vi "Do Action.vi"(8 "error in (no error)":errorcluster, 11 "Encoder Drive Straight in":refnum<class "Encoder Drive Straight.lvclass">) -> (0 "error out":errorcluster, 3 "Encoder Drive Straight out":refnum<class "Encoder Drive Straight.lvclass">)   [LabVIEW 2016, in "Encoder Drive Straight.lvclass"]
uses:
  Encoder Drive Straight.lvclass
  Encoder Drive Straight.lvclass/Encoder Drive Straight.ctl
panel:
  out "Waveform Chart":cluster{"Distance":dbl, "Encoder Target":dbl}(graph)
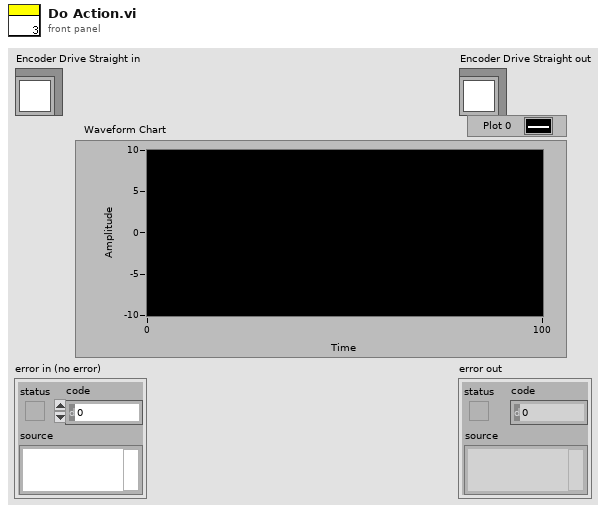
[diagram p1: front panel]
types:
  T1 = typedef "WPI_EncoderDevRef.ctl" = cluster{"DevStatus":errorcluster, "EncoderIndex":T2, "CounterIndex":T3, "DistancePerCount":dbl, "Decoding Type":T4}
  T2 = typedef "FPGA_EncoderIdx.ctl" = enum8{"Enc 0", "Enc 1", "Enc 2", "Enc 3", "Enc 4", "Enc 5", "Enc 6", "Enc 7", "Invalid"}
  T3 = typedef "FPGA_CounterCtrSystemIndex.ctl" = enum8{"Ctr 0", "Ctr 1", "Ctr 2", "Ctr 3", "Ctr 4", "Ctr 5", "Ctr 6", "Ctr 7", "Invalid"}
  T4 = typedef "WPI_EncoderType.ctl" = enum16{"1x", "2x", "4x"}
  T5 = typedef "WPI_RobotDriveDevRef.ctl" = cluster{"DevStatus":errorcluster, "Motors[]":T6[], "Square Inputs":bool, "Max Output":dbl}
  T6 = typedef "WPI_MotorControlDeviceRef.ctl" = cluster{"DeviceStatus":errorcluster, "Type":T7, "PWM":cluster{"PWM Channel":T8, "DeadBand":T9}, "CAN":cluster{"Device Number":u8, "SetOutput VI Ref":variant, "GetOutput VI Ref":variant, "Enable VI Ref":variant, "Disable VI Ref":variant, "Data":variant}, "Invert":bool}
  T7 = typedef "WPI_MotorControlType.ctl" = enum16{"PWM", "CAN"}
  T8 = typedef "FPGA_DIOPWMChannel.ctl" = enum8{"PWM 0", "PWM 1", "PWM 2", "PWM 3", "PWM 4", "PWM 5", "PWM 6", "PWM 7", "PWM 8", "PWM 9", "PWM MXP 0", "PWM MXP 1", "PWM MXP 2", "PWM MXP 3", "PWM MXP 4", "PWM MXP 5", "PWM MXP 6", "PWM MXP 7", "PWM MXP 8", "PWM MXP 9", "Invalid"}
  T9 = typedef "WPI_PWMDeadband.ctl" = cluster{"Name":string, "maxPositivePwm":i32, "minPositivePwm":i32, "centerPwm":i32, "maxNegativePwm":i32, "minNegativePwm":i32, "angularRange":u16}
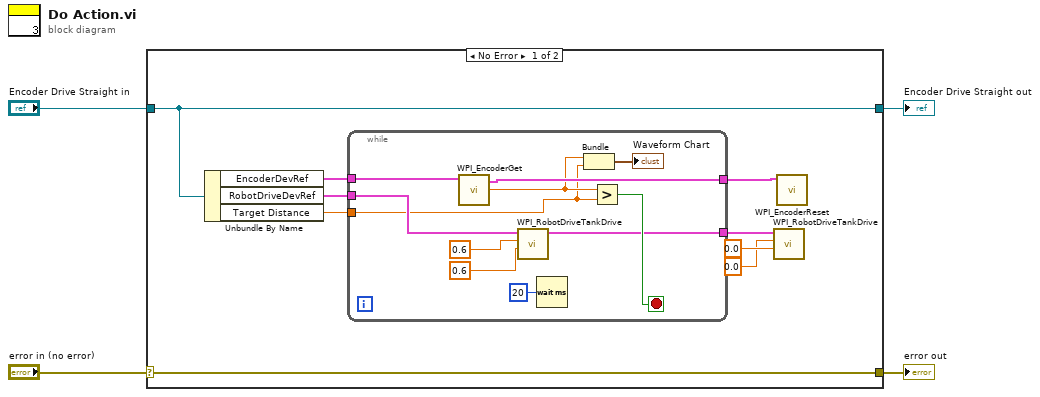
[diagram p0: block diagram]
diagram:
  n1 = case shown="No Error" "error in (no error)" {
    selector: "error in (no error)" -> [w13 w26]
    tunnel: [w13 w26] -> w3
    tunnel: [w12 w25] -> w1
    tunnel: "Encoder Drive Straight in" -> [w12 w25]
    frame No Error {
      n2 = Unbundle By Name(w12) -> ("EncoderDevRef"=w11:T1, "RobotDriveDevRef"=w10:T5, "Target Distance"=w5:dbl)
      n3 = while {
        tunnel: w11 -> [w24]
        tunnel: w10 -> [w23]
        tunnel: [w18] -> w9
        tunnel: [w17] -> w6
        tunnel: w5 -> [w14]
        stop <- w19 stop-if-true
        n4 = call <vilib>:"WPI_EncoderGet.vi"("EncoderDevRef"=w24) -> ("Distance"=w16:dbl, "EncoderDevRef"=w17:T1)  [unwired: 5 in, 4 out]
        n5 = call <vilib>:"WPI_RobotDriveTankDrive.vi"("Right axis value"=0.6, "Left axis value"=0.6, "RobotDriveDevRef"=w23) -> ("RobotDriveDevRef"=w18:T5)  [unwired: 6 in, 2 out]
        n6 = Wait (ms)(milliseconds to wait=u32 20) -> ()  [unwired: 1 out]
        n7 = Bundle("Distance"=w16, "Target Distance"=w14) -> (→"Waveform Chart":cluster{"Distance":dbl, "Target Distance":dbl})  [unwired: 1 in]
        n8 = Greater?(x=w16, y=w14) -> (0:w19:bool)
      }
      n9 = call <vilib>:"WPI_RobotDriveTankDrive.vi"("Right axis value"=0.0, "Left axis value"=0.0, "RobotDriveDevRef"=w9) -> ()  [unwired: 6 in, 3 out]
      n10 = call <vilib>:"WPI_EncoderReset.vi"("EncoderDevRef"=w6) -> ()  [unwired: 9 in, 2 out]
    }
    frame Error {
    }
  }
  "error out" <- w3
  "Encoder Drive Straight out" <- w1
